vi "Delete Element from Array (by ref) [U32].vi"(8 "Error In":errorcluster, 9 "Element Index":i32, 11 "Array in":refnum<vi>) -> (0 "Error Out":errorcluster, 1 "Array w/o Element at Index":u32[](array[numeric]), 3 "Array out":refnum<vi>)   [LabVIEW 2021, in "Arrays.lvlib"]
uses:
  Arrays.lvlib
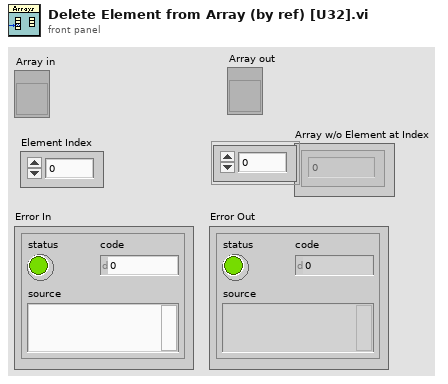
[diagram p1: front panel]
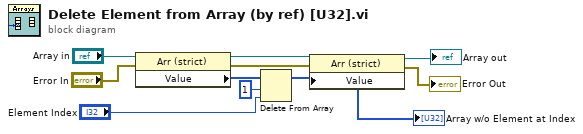
[diagram p0: block diagram]
diagram:
  n1 = property class="Arr (strict)"(reference="Array in", error in="Error In") -> (reference out=w9:refnum<vi>, error out=w6:errorcluster, "Value"=w8:u32[])
  n2 = Delete From Array(array=w8, length=1, index="Element Index") -> (array with subset deleted=w1:u32[])  [unwired: 1 out]
  "Array w/o Element at Index" <- w1
  n3 = property class="Arr (strict)"(reference=w9, error in=w6, "Value"=w1) -> (reference out=→"Array out":refnum<vi>, error out=→"Error Out":errorcluster)
